vi "main.vi"() -> ()   [LabVIEW 2020]
uses:
  <vilib>/Utility/file.llb/Write Delimited Spreadsheet (DBL).vi
  <vilib>/Utility/file.llb/Read Delimited Spreadsheet (DBL).vi
panel:
  out "Waveform Graph":dbl[](graph)
  out "Array":dbl[](array[numeric])
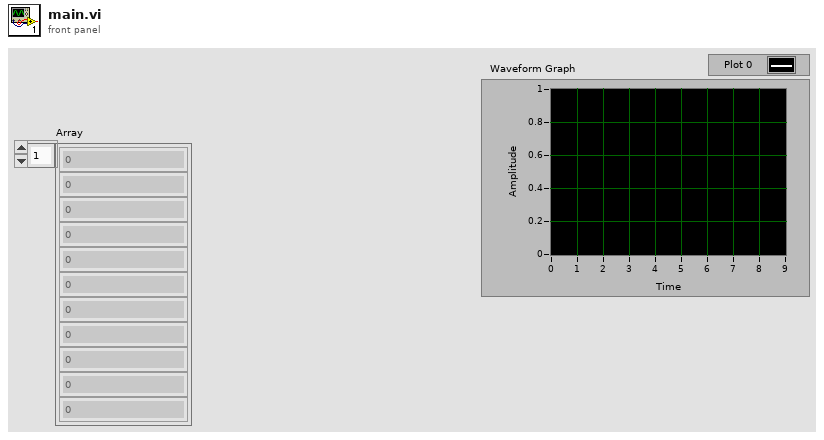
[diagram p1: front panel]
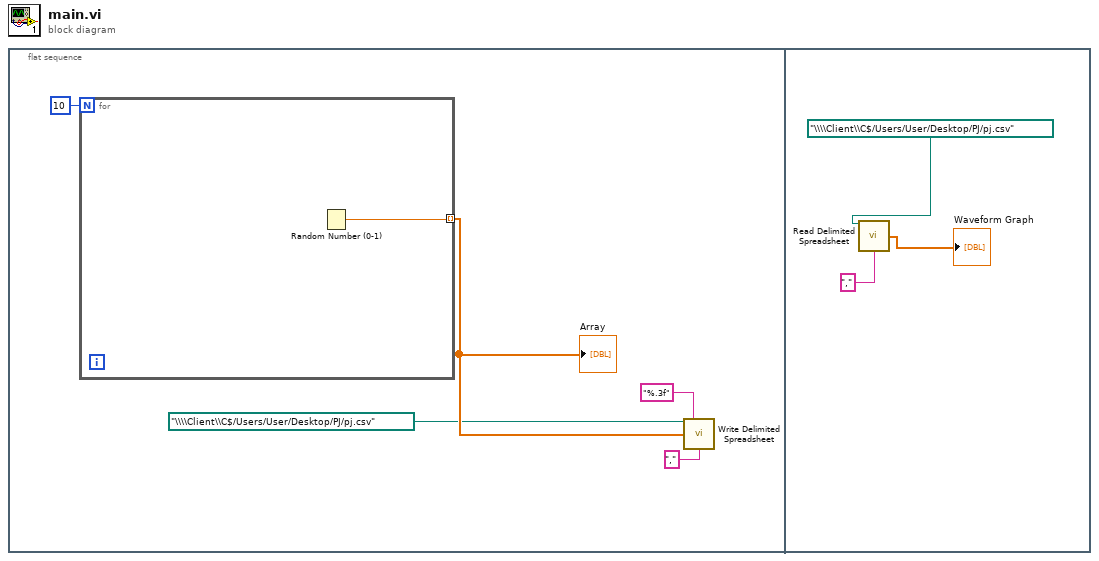
[diagram p0: block diagram]
diagram:
  n1 = flat-sequence {
    frame #0 {
      n2 = for {
        N: 10 -> [_]
        tunnel: [w6] -> w4 mode=indexing
        n3 = Random Number (0-1)() -> (number: 0 to 1=w6:dbl)
      }
      "Array" <- w4
      n4 = call-poly <vilib>:"Write Delimited Spreadsheet.vi"("file path (dialog if empty)"=path "\\\\Client\\C$/Users/User/Desktop/PJ/pj.csv", "format (%.3f)"="%.3f", "1D data"=w4, "delimiter (\\t)"="," ("delimiter (\\t)")) -> ()  [unwired: 10 in, 2 out]
    }
    frame #1 {
      n5 = call-poly <vilib>:"Read Delimited Spreadsheet.vi"("file path (dialog if empty)"=path "\\\\Client\\C$/Users/User/Desktop/PJ/pj.csv", "delimiter (\\t)"="," ("delimiter (\\t)")) -> ("first row"=→"Waveform Graph":dbl[])  [unwired: 8 in, 5 out]
    }
  }
